vi "Config Login.vi"(8 "error in (no error)":errorcluster, 11 "Configuration in":refnum<class "Configuration.lvclass">) -> (0 "error out":errorcluster, 3 "Configuration out":refnum<class "Configuration.lvclass">)   [LabVIEW 2016, in "Configuration.lvlib" / "Configuration.lvclass"]
uses:
  <userlib>/Configuration Dialog Actor/Configuration.lvclass
  C:/Program Files (x86)/National Instruments/LabVIEW 2016/vi.lib/ActorFramework/Actor/Actor.lvclass
  <userlib>/Configuration Dialog Actor/Configuration.lvclass/Configuration.ctl
  <vilib>/ActorFramework/Actor/Actor.lvclass/Actor.ctl
  <userlib>/Common Components/Function Messages/Log in MsgList Msg/Log in MsgList Msg.lvclass/Log in MsgList Msg.ctl
  <vilib>/ActorFramework/Message Enqueuer/Message Enqueuer.lvclass/Message Enqueuer.ctl
  <vilib>/ActorFramework/Message Enqueuer/Enqueue.vi
  <userlib>/Common Components/Function Messages/Log in MsgList Msg/Log in MsgList Msg.lvclass
  C:/Program Files (x86)/National Instruments/LabVIEW 2016/vi.lib/ActorFramework/Message/Message.lvclass
  <vilib>/ActorFramework/Message Priority Queue/Priority Enqueue.vi
  <userlib>/_OpenG.lib/md5/md5.llb/MD5 Message Digest (Hexadecimal String)__ogtk.vi
  <vilib>/ActorFramework/Actor/Actor.lvclass
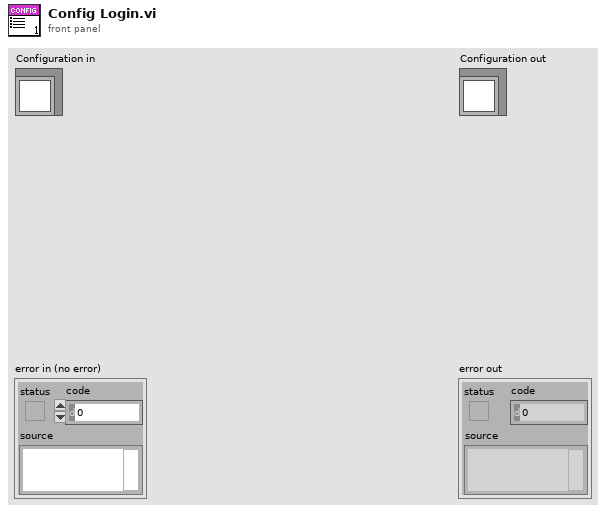
[diagram p1: front panel]
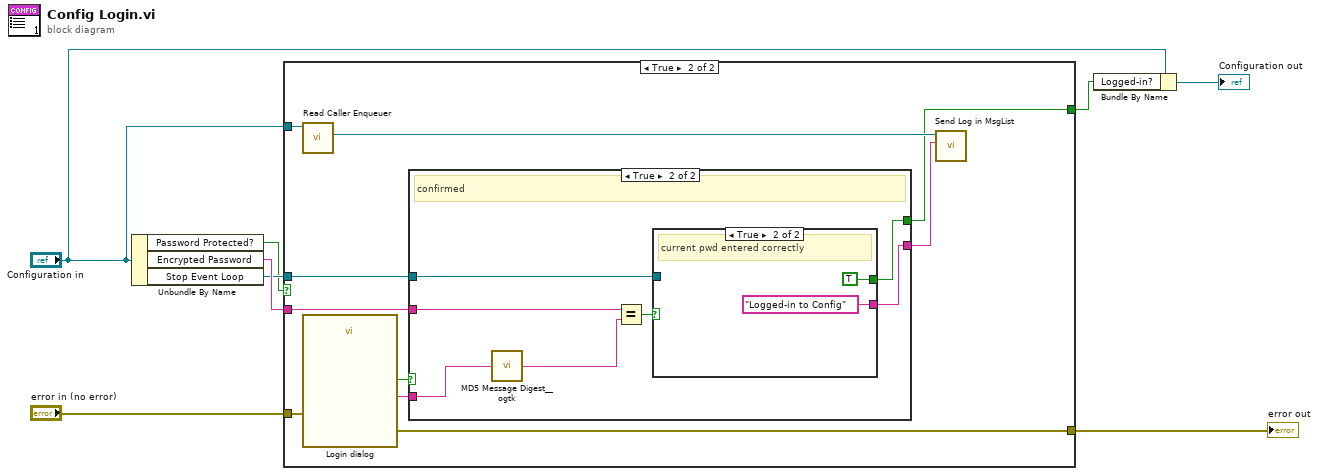
[diagram p0: block diagram]
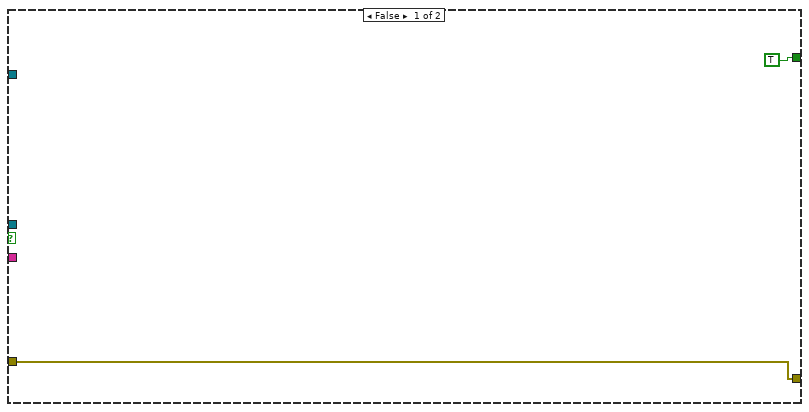
[diagram p2: hidden frame]
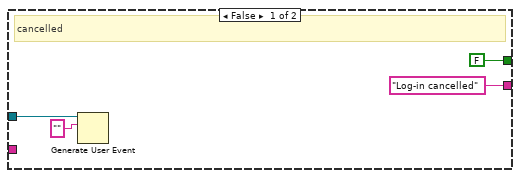
[diagram p3: hidden frame]
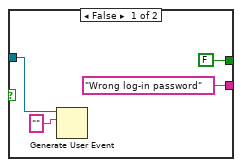
[diagram p4: hidden frame]
diagram:
  n1 = Unbundle By Name("Configuration in") -> ("Password Protected?"=w4:bool, "Encrypted Password"=w8:string, "Stop Event Loop"=w5:refnum<user-event>)
  n2 = case shown="True" w4 {
    tunnel: w8 -> [_ w18]
    tunnel: "error in (no error)" -> [w10 w15]
    tunnel: [w10 w14] -> w6
    tunnel: "Configuration in" -> [_ w13]
    tunnel: w5 -> [_ w12]
    tunnel: [TRUE w11] -> w1
    frame False {
    }
    frame True {
      n3 = call <vilib>:"Read Caller Enqueuer.vi"("Actor"=w13) -> ("Caller Enqueuer"=w17:refnum<class "Message Enqueuer.lvclass">)  [unwired: 10 in]
      n4 = call <userlib>:"Login dialog.vi"("error in (no error)"=w15) -> ("Admin log-in"=w19:string, "Confirm"=w20:bool, "error out"=w14:errorcluster)  [unwired: 16 in]
      n5 = case shown="True" w20 {
        tunnel: w19 -> [_ w31]
        tunnel: w18 -> [_ w30]
        tunnel: ["Log-in cancelled" ("Msg") w28] -> w16
        tunnel: w12 -> [w23 w27]
        tunnel: [FALSE w26] -> w11
        frame False {
          # "cancelled"
          n6 = Generate User Event(user event=w23, event data cluster="" ("event data")) -> ()  [unwired: 2 in, 2 out]
        }
        frame True {
          # "confirmed"
          n7 = call-poly <userlib>:"MD5 Message Digest__ogtk.vi"("Message"=w31) -> ("MD5 Message Digest"=w25:string)
          n8 = Equal?(x=w30, y=w25) -> (x = y?=w29:bool)
          n9 = case shown="True" w29 {
            tunnel: ["Wrong log-in password" "Logged-in to Config"] -> w28
            tunnel: w27 -> [w33 _]
            tunnel: [FALSE TRUE] -> w26
            frame False {
              n10 = Generate User Event(user event=w33, event data cluster="" ("event data")) -> ()  [unwired: 2 in, 2 out]
            }
            frame True {
              # "current pwd entered correctly"
            }
          }
        }
      }
      n11 = call <userlib>:"Send Log in MsgList.vi"("Msg"=w16, "Message Enqueuer"=w17) -> ()  [unwired: 8 in, 2 out]
    }
  }
  "error out" <- w6
  n12 = Bundle By Name(cluster="Configuration in", "Logged-in?"=w1) -> (→"Configuration out":refnum<class "Configuration.lvclass">)
